vi "Cargar USD.vi"(7 "USD Actor.lvlib:USD Actor.lvclass":refnum<class "USD Actor.lvclass">) -> (5 "USD Actor.lvlib:USD Actor.lvclass 2":refnum<class "USD Actor.lvclass">)   [LabVIEW 2019, in "USD Actor.lvlib" / "USD Actor.lvclass"]
uses:
  USD Actor.lvclass
  USD Actor.lvclass/USD Actor.ctl
  <vilib>/Utility/config.llb/Read Key (String).vi
  <vilib>/Utility/config.llb/NI_LVConfig.lvlib
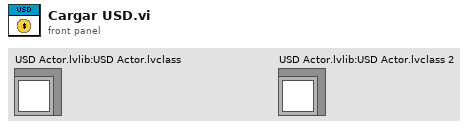
[diagram p1: front panel]
types:
  T1 = typedef "NI_LVConfig.lvlib/Config Data RefNum.ctl" = refnum<k1>
  T2 = cluster{"[0]":string, "[1]":string, "[2]":string, "[3]":string, "[4]":string, "[5]":string, "[6]":string, "[7]":string, "[8]":string}
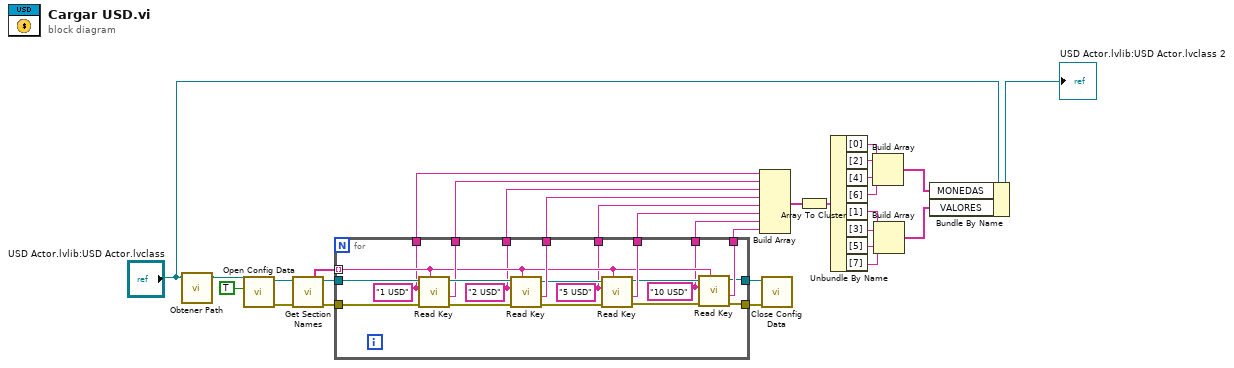
[diagram p0: block diagram]
diagram:
  n1 = call "Obtener Path.vi"("USD Actor.lvlib:USD Actor.lvclass"="USD Actor.lvlib:USD Actor.lvclass") -> ("appended path"=w2:path)  [unwired: 10 in]
  n2 = call <vilib>:"Open Config Data.vi"("create file if necessary (T)"=TRUE, "configuration file path"=w2) -> ("error out"=w30:errorcluster, "refnum"=w29:T1)  [unwired: 7 in, 1 out]
  n3 = call <vilib>:"Get Section Names.vi"("error in (no error)"=w30, "refnum"=w29) -> ("error out"=w27:errorcluster, "section names"=w24:string[], "refnum out"=w28:T1)  [unwired: 7 in]
  n4 = for {
    tunnel: w28 -> [w50]
    tunnel: w27 -> [w49]
    tunnel: w24 -> [w36] mode=indexing
    tunnel: [w40] -> w26
    tunnel: [w41] -> w25
    tunnel: [w47] -> w22
    tunnel: [w46] -> w20
    tunnel: [w45] -> w18
    tunnel: [w44] -> w16
    tunnel: [w35] -> w23
    tunnel: [w34] -> w21
    tunnel: [w33] -> w19
    tunnel: [w32] -> w17
    w32 = "10 USD" ("key")
    w33 = "5 USD" ("key")
    w34 = "2 USD" ("key")
    w35 = "1 USD" ("key")
    n5 = call-poly <vilib>:"Read Key.vi"("section"=w36, "error in (no error)"=w49, "key"=w35, "refnum"=w50) -> ("error out"=w37:errorcluster, "value"=w47:string, "refnum out"=w48:T1)  [unwired: 4 in, 1 out]
    n6 = call-poly <vilib>:"Read Key.vi"("section"=w36, "error in (no error)"=w37, "key"=w34, "refnum"=w48) -> ("error out"=w38:errorcluster, "value"=w46:string, "refnum out"=w42:T1)  [unwired: 4 in, 1 out]
    n7 = call-poly <vilib>:"Read Key.vi"("section"=w36, "error in (no error)"=w38, "key"=w33, "refnum"=w42) -> ("error out"=w39:errorcluster, "value"=w45:string, "refnum out"=w43:T1)  [unwired: 4 in, 1 out]
    n8 = call-poly <vilib>:"Read Key.vi"("section"=w36, "error in (no error)"=w39, "key"=w32, "refnum"=w43) -> ("error out"=w40:errorcluster, "value"=w44:string, "refnum out"=w41:T1)  [unwired: 4 in, 1 out]
  }
  n9 = Build Array(w23, w22, w21, w20, w19, w18, w17, w16) -> (w15:string[])
  n10 = call <vilib>:"Close Config Data.vi"("error in (no error)"=w26, "refnum"=w25) -> ()  [unwired: 8 in, 2 out]
  n11 = Array To Cluster(array=w15) -> (cluster=w14:T2)
  n12 = Unbundle By Name(w14) -> ("[0]"=w10:string, "[2]"=w13:string, "[4]"=w11:string, "[6]"=w12:string, "[1]"=w9:string, "[3]"=w8:string, "[5]"=w7:string, "[7]"=w6:string)
  n13 = Build Array(w10, w13, w11, w12) -> (w4:string[])
  n14 = Build Array(w9, w8, w7, w6) -> (w5:string[])
  n15 = Bundle By Name(cluster="USD Actor.lvlib:USD Actor.lvclass", "MONEDAS"=w4, "VALORES"=w5) -> (→"USD Actor.lvlib:USD Actor.lvclass 2":refnum<class "USD Actor.lvclass">)
